vi "update-signal-names.vi"(8 "error in (no error)":errorcluster, 9 "frame.tag":string, 11 "dbc in":refnum<class "dbc.lvclass">) -> (0 "error out":errorcluster, 3 "dbc out":refnum<class "dbc.lvclass">)   [LabVIEW 2015, in "dbc.lvclass"]
uses:
  dbc.lvclass
  controls/signal.result.ctl
  dbc.lvclass/dbc.ctl
  class.can.table/bAPPdata.lvclass
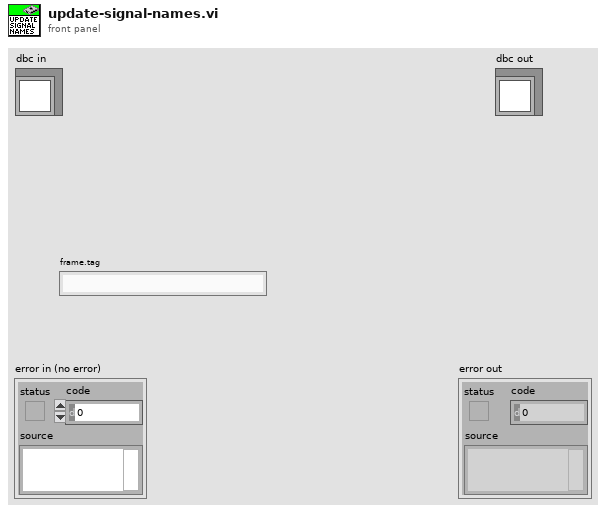
[diagram p1: front panel]
types:
  T1 = typedef "signal.result.ctl" = cluster{"Signal name":string, "payload":u8}
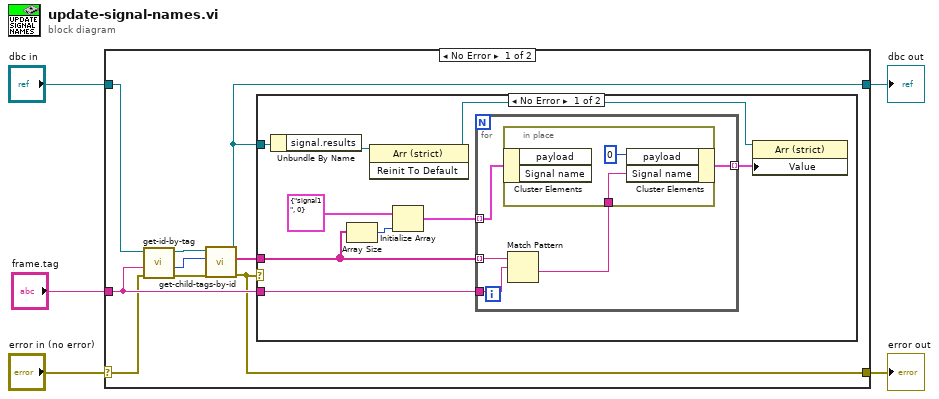
[diagram p0: block diagram]
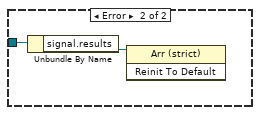
[diagram p2: hidden frame]
diagram:
  n1 = case shown="No Error" "error in (no error)" {
    selector: "error in (no error)" -> [w7 w34]
    tunnel: [w6 w34] -> w4
    tunnel: [w12 w33] -> w2
    tunnel: "dbc in" -> [w13 w33]
    tunnel: "frame.tag" -> [w9 _]
    frame No Error {
      n2 = call "get-id-by-tag.vi"("error in (no error)"=w7, "tag"=w9, "CANtable in"=w13) -> ("error out"=w8:errorcluster, "id"=w10:u32, "CANtable out"=w11:refnum<class "dbc.lvclass">)  [unwired: 6 in]
      n3 = call "get-child-tags-by-id.vi"("error in (no error)"=w8, "id"=w10, "CANtable in"=w11) -> ("error out"=w6:errorcluster, "child.rags"=w14:string[], "CANtable out"=w12:refnum<class "dbc.lvclass">)  [unwired: 6 in]
      n4 = case shown="No Error" w6 {
        tunnel: w14 -> [w17 _]
        tunnel: w12 -> [w16 w31]
        tunnel: w9 -> [w15 _]
        frame No Error {
          n5 = Unbundle By Name(w16) -> ("signal.results"=w23:refnum<vi>)
          n6 = Array Size(array=w17) -> (size(s)=w19:i32)
          n7 = invoke class="Arr (strict)" method="Reinit To Default"(reference=w23) -> (reference out=w22:refnum<vi>)  [unwired: 2 in, 2 out]
          n8 = Initialize Array(T1 {"Signal name"="signal1", "payload"=0} ("signal.results"), w19) -> (w18:T1[])
          n9 = for {
            tunnel: [w28] -> w21 mode=indexing
            tunnel: w17 -> [w26] mode=indexing
            tunnel: w18 -> [w27] mode=indexing
            tunnel: w15 -> [w25]
            n10 = Match Pattern(string=w26, regular expression=w25) -> (after substring=w24:string)  [unwired: 1 in, 3 out]
            n11 = in-place {
              in-place-border: w24 -> [w29]
              n12 = in-place-cluster #1(w27) -> ()  [unwired: 2 out]
              n13 = in-place-cluster #1("payload"=0, "Signal name"=w29) -> (w28:T1)
            }
          }
          n14 = property class="Arr (strict)"(reference=w22, "Value"=w21) -> ()  [unwired: 1 in, 2 out]
        }
        frame Error {
          n15 = Unbundle By Name(w31) -> ("signal.results"=w32:refnum<vi>)
          n16 = invoke class="Arr (strict)" method="Reinit To Default"(reference=w32) -> ()  [unwired: 2 in, 3 out]
        }
      }
    }
    frame Error {
    }
  }
  "error out" <- w4
  "dbc out" <- w2
